vi "Expert_NumAvailableDevices.vi"(11 "Error IN LabVIEW":errorcluster) -> (4 "numAvailablesCUDADevices":i32, 15 "Error OUT LabVIEW":errorcluster)   [LabVIEW 2018]
doc: "It indicates the number of GPU devices compatible with CUDA that the device has."
uses:
  dll/LibreriaAutis_3.dll
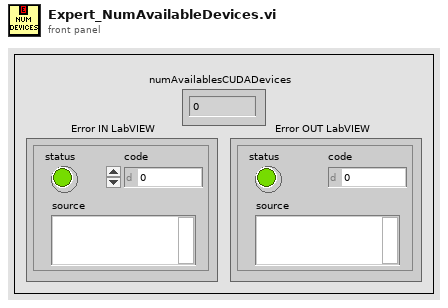
[diagram p1: front panel]
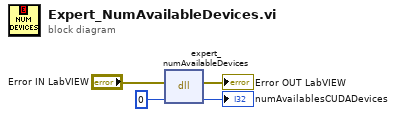
[diagram p0: block diagram]
diagram:
  n1 = dll-call lib="C:/Users/AUTIS/Desktop/LibreriaAUTIS/LabVIEW/dll/LibreriaAutis_3.dll" fn="expert_numAvailableDevices"(error in="Error IN LabVIEW", "numCUDADevices"=0) -> (error out=→"Error OUT LabVIEW":errorcluster, "numCUDADevices"=→"numAvailablesCUDADevices":i32)  [unwired: 3 in, 1 out]
